vi "Verify run direction.vi"(1 "Source":T1, 3 "Type&direction IN":T2) -> (0 "Type&direction OUT":T2)   [LabVIEW 2019, in "Exaprom PDF.lvlib"]
uses:
  Controls/Text Controls/Unicode/Type and run direction.ctl
  Controls/Text Controls/Unicode/Source rub direction.ctl
  Exaprom PDF.lvlib
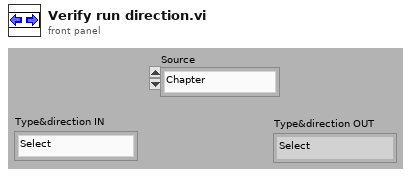
[diagram p1: front panel]
types:
  T1 = typedef "Exaprom PDF.lvlib/Source rub direction.ctl" = enum16{"Chapter", "Paragraph", "Phrase", "pdfpcell"}
  T2 = typedef "Exaprom PDF.lvlib/Type and run direction.ctl" = enum16{"Select", "ASCII", "UTF-16", "UTF-16 (default)", "UTF-16 (LTR)", "UTF-16 (RTL)"}
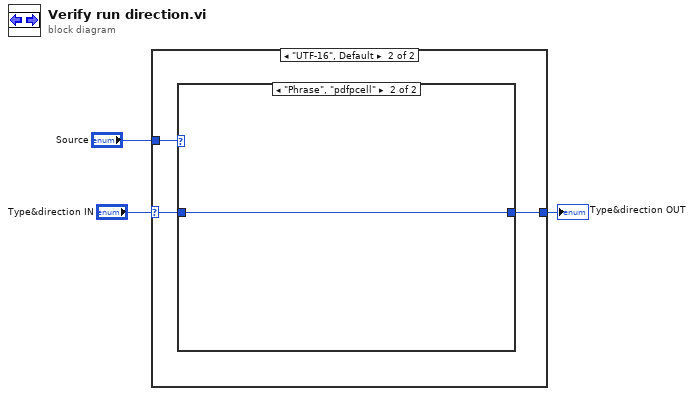
[diagram p0: block diagram]
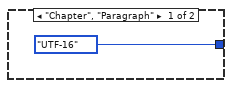
[diagram p3: hidden frame]
diagram:
  n1 = case shown="\"UTF-16\", Default" "Type&direction IN" {
    selector: "Type&direction IN" -> [w4 w5]
    tunnel: "Source" -> [_ w7]
    tunnel: [w4 w6] -> w1
    frame "ASCII" {
    }
    frame "UTF-16", Default {
      n2 = case shown="\"Phrase\", \"pdfpcell\"" w7 {
        tunnel: [Type_and_run_direction."UTF-16" ("Type&direction OUT") w9] -> w6
        tunnel: w5 -> [_ w9]
        frame "Chapter", "Paragraph" {
        }
        frame "Phrase", "pdfpcell" {
        }
      }
    }
  }
  "Type&direction OUT" <- w1
